vi "sub_read_wav.vi"(11 "file path (use dialog)":path) -> (0 "sound format":T1={"sample rate (S/s)"=22050.0, "number of channels"=2, "bits per sample"=16}, 3 "I16 sound data":i16[](array[numeric]))   [LabVIEW 2014]
uses:
  <vilib>/sound2/lvsound2.llb/Sound Data Format.ctl
  <vilib>/sound2/lvsound2.llb/Sound File Position.ctl
  <vilib>/sound2/lvsound2.llb/Sound File Info (path).vi
panel:
  out "element":waveform(dbl)
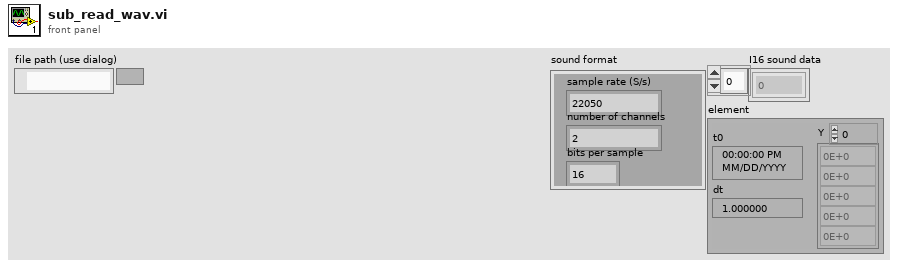
[diagram p1: front panel]
types:
  T1 = typedef "Sound Data Format.ctl" = cluster{"sample rate (S/s)":dbl, "number of channels":i32, "bits per sample":i32}
  T2 = typedef "Sound File Position.ctl" = u16
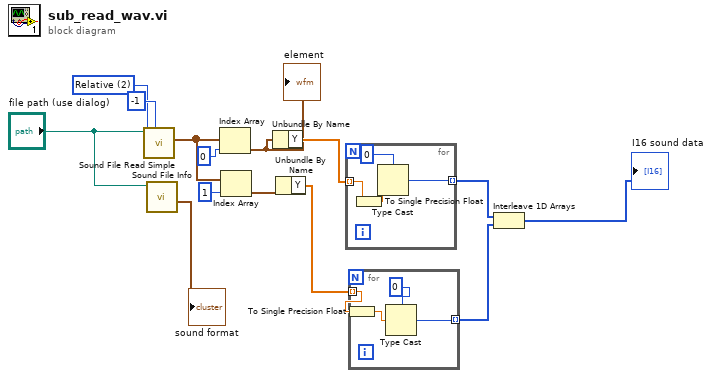
[diagram p0: block diagram]
diagram:
  w11 = T2 2 items=["Absolute"=0, "Relative"=2] ("position mode")
  n1 = call <vilib>:"Sound File Read Simple.vi"("number of samples/ch (-1: all)"=-1, "position mode"=w11, "path"="file path (use dialog)") -> ("data"=w10:waveform(dbl)[])  [unwired: 5 in, 3 out]
  n2 = call-poly <vilib>:"Sound File Info.vi"("path"="file path (use dialog)") -> ("sound format"=→"sound format":T1)  [unwired: 7 in, 3 out]
  n3 = Index Array(array=w10, index=0) -> (element=w1:waveform(dbl))
  "element" <- w1
  n4 = Index Array(array=w10, index=1) -> (element=w7:waveform(dbl))
  n5 = Unbundle By Name(w1) -> ("Y"=w6:dbl[])
  n6 = Unbundle By Name(w7) -> ("Y"=w5:dbl[])
  n7 = for {
    tunnel: w6 -> [w16] mode=indexing
    tunnel: [w17] -> w3 mode=indexing
    n8 = To Single Precision Float(number=w16) -> (single precision float=w15:sgl)
    n9 = Type Cast(type=i16 0, x=w15) -> (*(type *) &x=w17:i16)
  }
  n10 = for {
    tunnel: w5 -> [w20] mode=indexing
    tunnel: [w21] -> w4 mode=indexing
    n11 = To Single Precision Float(number=w20) -> (single precision float=w19:sgl)
    n12 = Type Cast(type=i16 0, x=w19) -> (*(type *) &x=w21:i16)
  }
  n13 = Interleave 1D Arrays(w3, w4) -> (→"I16 sound data":i16[])
